vi "Unload.vi"(0 "LV MDI in":refnum<class "LV MDI.lvclass">, 5 "Doc Name[]":string[](array[string]), 11 "error in (no error)":errorcluster) -> (4 "LV MDI out":refnum<class "LV MDI.lvclass">, 6 "Doc Name out[]":string[](array[string]), 15 "error out":errorcluster)   [LabVIEW 2016, in "LV MDI.lvclass"]
doc: "Unload Documents from memory"
uses:
  LV MDI.lvclass
  LV MDI.lvclass/LV MDI.ctl
  Document/Document.lvclass/Document.ctl
  user32.dll
  Document/Document.lvclass
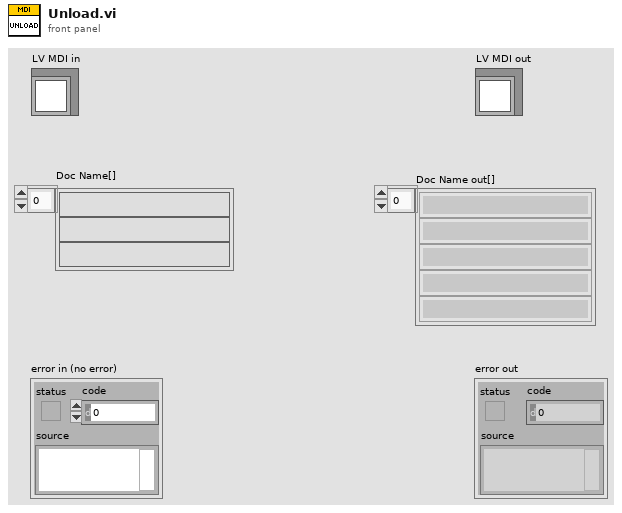
[diagram p1: front panel]
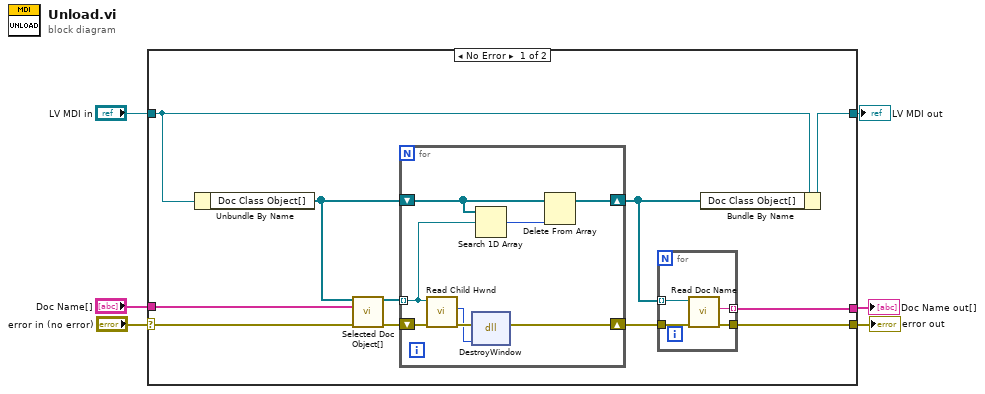
[diagram p0: block diagram]
diagram:
  n1 = case shown="No Error" "error in (no error)" {
    selector: "error in (no error)" -> [w15 w31]
    tunnel: [w9 w31] -> w5
    tunnel: [w17 w30] -> w3
    tunnel: "LV MDI in" -> [w16 w30]
    tunnel: "Doc Name[]" -> [w11 _]
    tunnel: [w7 _] -> w1
    frame No Error {
      n2 = Unbundle By Name(w16) -> ("Doc Class Object[]"=w13:refnum<class "Document.lvclass">[])
      n3 = call "Selected Doc Object[].vi"("Doc Class Object[]"=w13, "Doc Name[]"=w11, "error in"=w15) -> ("Selected Doc[]"=w12:refnum<class "Document.lvclass">[], "error Out"=w14:errorcluster)  [unwired: 11 in]
      n4 = for {
        shift-right: [w24] -> w10
        shift-left: w14 -> [w29]
        tunnel: w12 -> [w22] mode=indexing
        shift-right: [w23] -> w8
        shift-left: w13 -> [w26]
        n5 = call "Read Child Hwnd.vi"("error in (no error)"=w29, "Document in"=w22) -> ("error out"=w28:errorcluster, "Child Hwnd"=w27:u32)  [unwired: 7 in, 1 out]
        n6 = dll-call lib="user32.dll" fn="DestroyWindow"(error in=w28, "hwnd"=w27) -> (error out=w24:errorcluster)  [unwired: 4 in, 1 out]
        n7 = Search 1D Array(1D array=w26, element=w22) -> (index of element=w25:i32)  [unwired: 1 in]
        n8 = Delete From Array(array=w26, index=w25) -> (array with subset deleted=w23:refnum<class "Document.lvclass">[])  [unwired: 1 in, 1 out]
      }
      n9 = for {
        tunnel: [w20] -> w9
        tunnel: w10 -> [w21]
        tunnel: w8 -> [w19] mode=indexing
        tunnel: [w18] -> w7 mode=indexing
        n10 = call "Read Doc Name.vi"("error in (no error)"=w21, "Document in"=w19) -> ("error out"=w20:errorcluster, "Doc Name"=w18:string)  [unwired: 7 in, 1 out]
      }
      n11 = Bundle By Name(cluster=w16, "Doc Class Object[]"=w8) -> (w17:refnum<class "LV MDI.lvclass">)
    }
    frame Error {
    }
  }
  "error out" <- w5
  "LV MDI out" <- w3
  "Doc Name out[]" <- w1
